vi "z_0__v1.vi"(9 "y[0]":ext, 10 "x[0]":ext, 11 "R":ext) -> (3 "z[0]":ext)   [LabVIEW 2020]
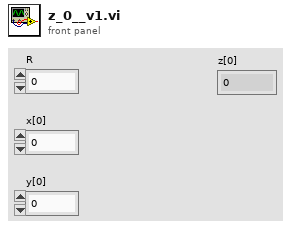
[diagram p1: front panel]
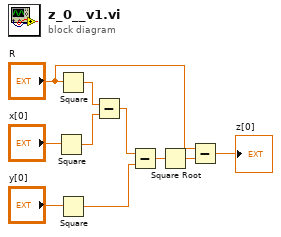
[diagram p0: block diagram]
diagram:
  n1 = Square(x="x[0]") -> (x^2=w7:ext)
  n2 = Square(x="R") -> (x^2=w8:ext)
  n3 = Square(x="y[0]") -> (x^2=w5:ext)
  n4 = Subtract(x=w8, y=w7) -> (x-y=w6:ext)
  n5 = Subtract(x=w6, y=w5) -> (x-y=w4:ext)
  n6 = Square Root(x=w4) -> (sqrt(x)=w3:ext)
  n7 = Subtract(x="R", y=w3) -> (x-y=→"z[0]":ext)
